vi "ReadFromFile.vi"(4 "Sequence Context":T1) -> (0 "error out":errorcluster, 1 "Test Data":T2 {"Numeric Measurement" format="%.2f"})   [LabVIEW 2013]
uses:
  <vilib>/addons/TestStand/_TSLegacy.llb/LabVIEW Test - Test Data.ctl
  <vilib>/addons/TestStand/_TSLegacy.llb/LabVIEW Test - Sequence Context.ctl
panel:
  out "Data Read":string
  in  "File Refnum":refnum<file>
  in  "Boolean":bool
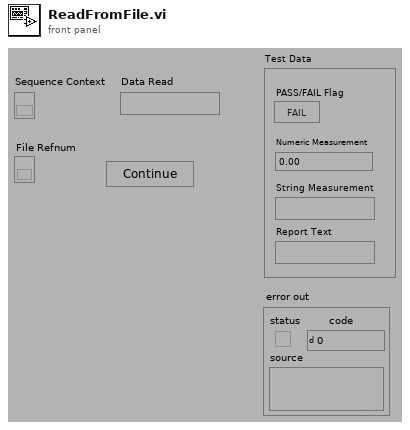
[diagram p1: front panel]
types:
  T1 = typedef "LabVIEW Test - Sequence Context.ctl" = refnum<k7>
  T2 = typedef "LabVIEW Test - Test Data.ctl" = cluster{"PASS/FAIL Flag":bool, "Numeric Measurement":dbl, "String Measurement":string, "Report Text":string}
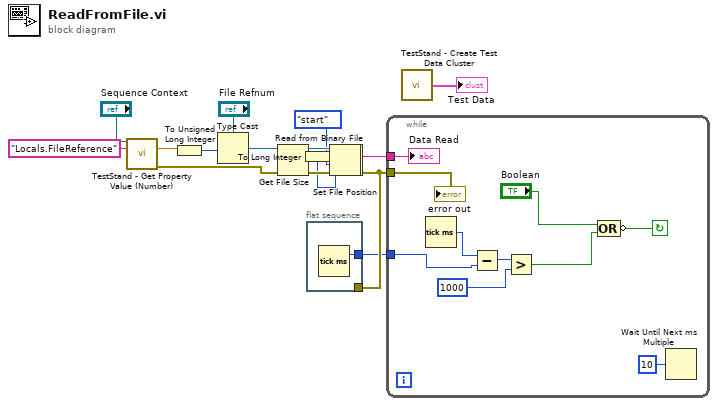
[diagram p0: block diagram]
diagram:
  n1 = call <vilib>:"TestStand - Get Property Value (Number).vi"("Sequence Context In"="Sequence Context", "Lookup String"="Locals.FileReference") -> ("Value"=w8:dbl, "error out"=w13:errorcluster)  [unwired: 1 in, 11 out]
  n2 = To Unsigned Long Integer(number=w8) -> (unsigned 32bit integer=w7:u32)
  n3 = Type Cast(type="File Refnum", x=w7) -> (*(type *) &x=w15:refnum<file>)
  n4 = Get File Size(file=w15, error in=w13) -> (refnum out=w14:refnum<file>, size (in bytes)=w3:i64, 0:w12:errorcluster)
  n5 = To Long Integer(number=w3) -> (32bit integer=w11:i32)
  n6 = flat-sequence {
    tunnel: [w19] -> w4
    tunnel: w5 -> [_]
    frame #0 {
      n7 = Tick Count (ms)() -> (millisecond timer value=w19:u32)
    }
  }
  n8 = Set File Position(refnum=w14, from (0:start)=enum16{"start", "end", "current"}."start" ("pos mode (0:2)"), error in=w12) -> (refnum out=w2:refnum<file>, error out=w1:errorcluster)  [unwired: 1 out]
  n9 = Read from Binary File(8:w1, 10:w11, 11:w2) -> (0:w5:errorcluster, 2:w9:string)  [unwired: 5 out]
  n10 = while {
    tunnel: w5 -> [w28]
    tunnel: w9 -> [w29]
    tunnel: w4 -> [w24]
    stop <- w20 continue-if-true
    n11 = Tick Count (ms)() -> (millisecond timer value=w25:u32)
    n12 = Subtract(x=w25, y=w24) -> (x-y=w26:u32)
    n13 = Greater?(x=w26, y=u32 1000) -> (0:w21:bool)
    n14 = Compound Arithmetic op=OR("Boolean", w21) -> (invert w20:bool)
    n15 = Wait Until Next ms Multiple(millisecond multiple=u32 10) -> ()  [unwired: 1 out]
    "error out" <- w28
    "Data Read" <- w29
  }
  n16 = call <vilib>:"TestStand - Create Test Data Cluster.vi"() -> ("Test Data"=→"Test Data":T2)  [unwired: 4 in]
